vi "Get Self Attributes.vi"(11 "Base Sender in":refnum<class "Base Sender.lvclass">) -> (2 "Self Attributes":refnum<class "Attributes.lvclass">)   [LabVIEW 2020, in "jettl.lvlib" / "Sender.lvlib" / "Base Sender.lvclass"]
uses:
  Base Sender.lvclass
  Attributes/Attributes/Attributes.lvclass
  Base Sender.lvclass/Base Sender.ctl
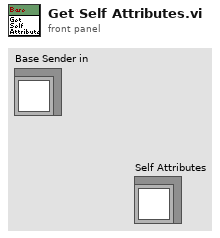
[diagram p1: front panel]
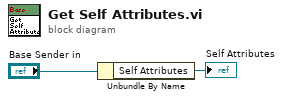
[diagram p0: block diagram]
diagram:
  n1 = Unbundle By Name("Base Sender in") -> ("Self Attributes"=→"Self Attributes":refnum<class "Attributes.lvclass">)
